vi "niFpga wdp fft streaming control chain.vi"(6 "enable":bool, 8 "enable 1":bool, 11 "input frame start":bool) -> (0 "frame start":bool, 1 "index=0?":bool, 2 "switch":bool[](array[boolean]), 3 "twiddle factors 1":T1(array[cluster]), 5 "twiddle factors":T1(array[cluster]))   [LabVIEW 2017]
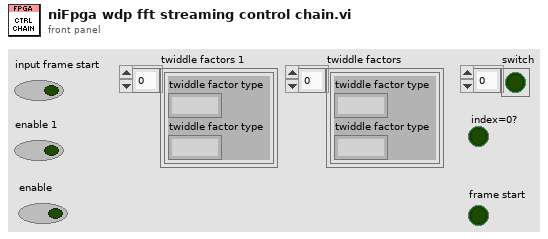
[diagram p1: front panel]
types:
  T1 = cluster{"twiddle factor type":fxp<+/-,16,2>, "twiddle factor type":fxp<+/-,16,2>}[]
  T2 = cluster{"twiddle factor type":fxp<+/-,16,2>, "twiddle factor type":fxp<+/-,16,2>}
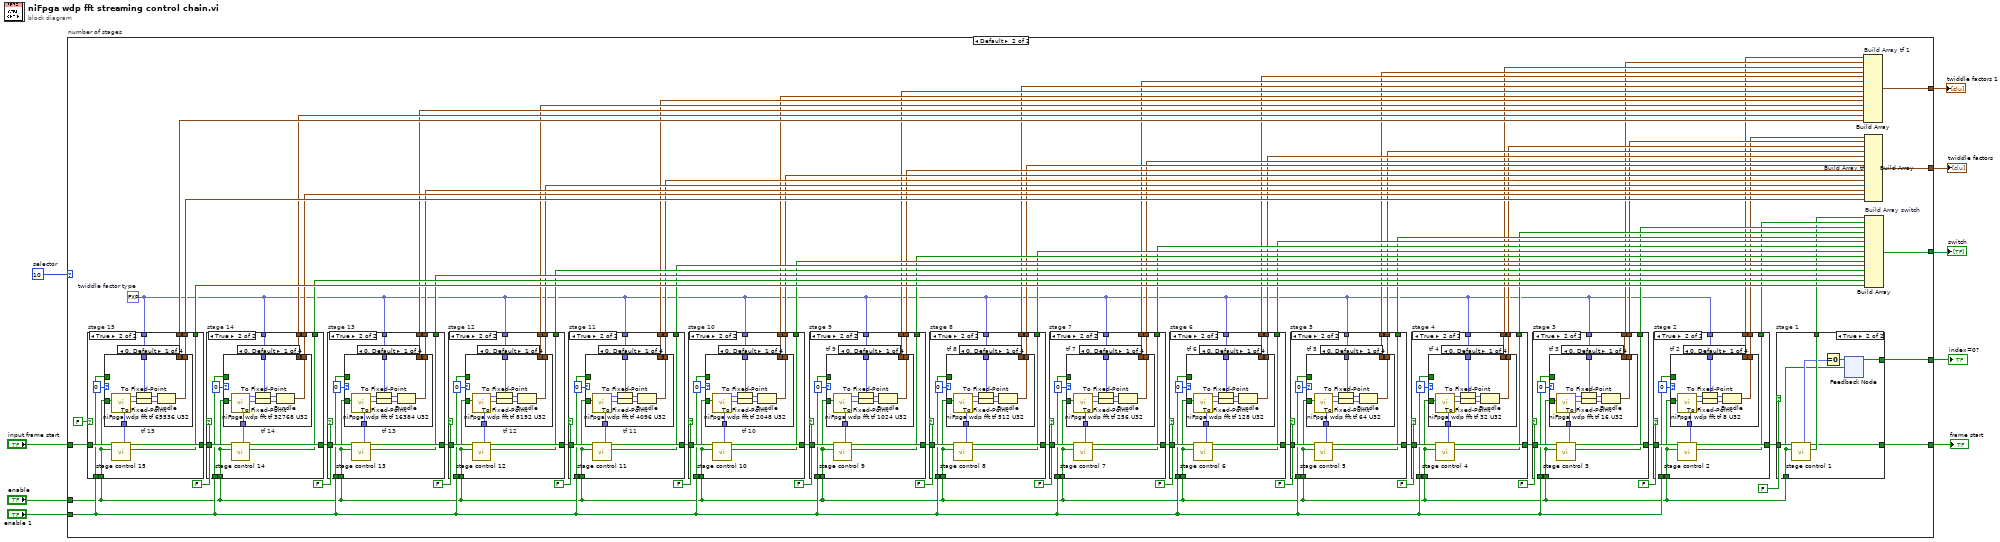
[diagram p0: block diagram]
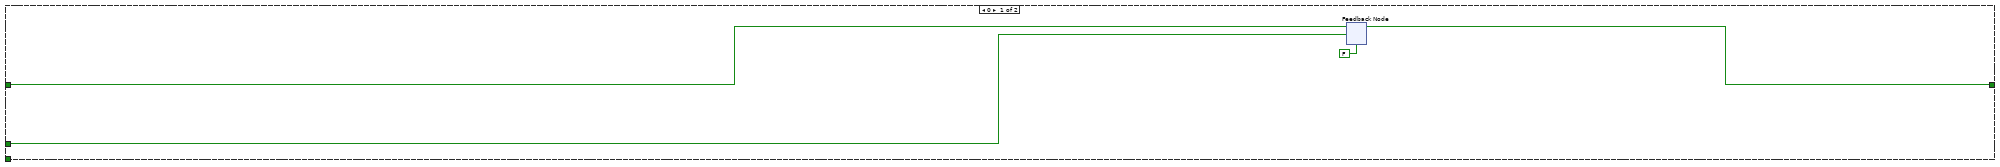
[diagram p2: hidden frame]
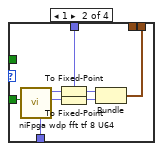
[diagram p5: hidden frame]
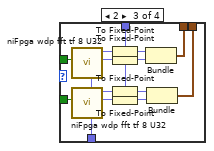
[diagram p6: hidden frame]
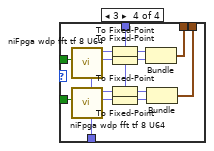
[diagram p7: hidden frame]
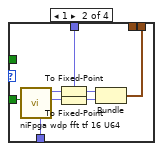
[diagram p9: hidden frame]
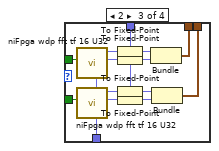
[diagram p10: hidden frame]
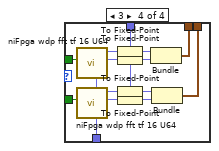
[diagram p11: hidden frame]
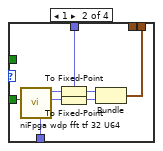
[diagram p13: hidden frame]
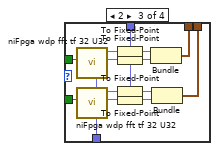
[diagram p14: hidden frame]
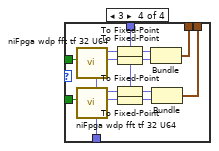
[diagram p15: hidden frame]
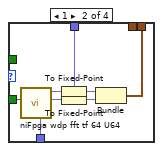
[diagram p17: hidden frame]
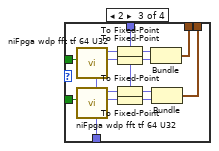
[diagram p18: hidden frame]
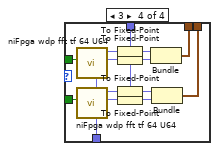
[diagram p19: hidden frame]
diagram:
  w2 = u8 10  # selector
  n1 = case "number of stages" shown="Default" w2 {
    tunnel: [_ w94] -> w9
    tunnel: [_ w93] -> w8
    tunnel: [_ w92] -> w7
    tunnel: "input frame start" -> [w12 w91]
    tunnel: [w11 w14] -> w5
    tunnel: "enable" -> [w10 w17]
    tunnel: "enable 1" -> [_ w35]
    tunnel: [_ w32] -> w1
    frame 0 {
      n2 = feedback #1(FALSE ("input frame start")) -> (w11:bool)
      n3 = feedback-in #1(w12, w10) -> ()
    }
    frame Default {
      w16 = fxp<+/-,16,2> 0.0  # twiddle factor type
      n4 = case "stage 15" shown="True" FALSE {
        tunnel: w91 -> [w818 w828]
        tunnel: [w818 w827] -> w87
        tunnel: w17 -> [_ w826]
        tunnel: w35 -> [_ w825]
        tunnel: [_ w824] -> w90
        tunnel: [_ w823] -> w89
        tunnel: [_ w822] -> w88
        tunnel: w16 -> [_ w819]
        frame False {
        }
        frame True {
          n5 = call "stage control 15"("enable"=w826, "frame start in"=w828) -> ("next switch"=w822:bool, "frame start out"=w827:bool, "twid index"=w820:fxp<+,15,15>)  [unwired: 7 in]
          n6 = case "tf 15" shown="0, Default" i16 0 {
            tunnel: w819 -> [w830 w838 w854 w868]
            tunnel: w826 -> [w834 w842 w853 w867]
            tunnel: w825 -> [_ _ w852 w866]
            tunnel: [_ _ w847 w861] -> w824
            tunnel: [w831 w839 w846 w860] -> w823
            tunnel: w820 -> [w829 w837 w845 w859]
            frame 0, Default {
              n7 = call <vilib>:"niFpga wdp fft tf 65536 U32.vi"("index"=w829, "enable"=w834) -> ("imag"=w835:fxp<+/-,16,2>, "real"=w836:fxp<+/-,16,2>)  [unwired: 8 in]
              n8 = To Fixed-Point(fixed-point type=w830, number=w836) -> (fixed-point=w833:fxp<+/-,16,2>)
              n9 = To Fixed-Point(fixed-point type=w830, number=w835) -> (fixed-point=w832:fxp<+/-,16,2>)
              n10 = Bundle("twiddle factor type"=w833, "twiddle factor type"=w832) -> (w831:T2)  [unwired: 1 in]
            }
            frame 1 {
              n11 = call <vilib>:"niFpga wdp fft tf 65536 U64.vi"("index"=w837, "enable"=w842) -> ("imag"=w843:fxp<+/-,32,2>, "real"=w844:fxp<+/-,32,2>)  [unwired: 8 in]
              n12 = To Fixed-Point(fixed-point type=w838, number=w844) -> (fixed-point=w841:fxp<+/-,16,2>)
              n13 = To Fixed-Point(fixed-point type=w838, number=w843) -> (fixed-point=w840:fxp<+/-,16,2>)
              n14 = Bundle("twiddle factor type"=w841, "twiddle factor type"=w840) -> (w839:T2)  [unwired: 1 in]
            }
            frame 2 {
              n15 = call <vilib>:"niFpga wdp fft tf 65536 U32.vi"("index"=w845, "enable"=w852) -> ("imag"=w856:fxp<+/-,16,2>, "real"=w857:fxp<+/-,16,2>)  [unwired: 8 in]
              n16 = call <vilib>:"niFpga wdp fft tf 65536 U32.vi"("index"=w845, "enable"=w853) -> ("imag"=w855:fxp<+/-,16,2>, "real"=w858:fxp<+/-,16,2>)  [unwired: 8 in]
              n17 = To Fixed-Point(fixed-point type=w854, number=w857) -> (fixed-point=w851:fxp<+/-,16,2>)
              n18 = To Fixed-Point(fixed-point type=w854, number=w856) -> (fixed-point=w850:fxp<+/-,16,2>)
              n19 = To Fixed-Point(fixed-point type=w854, number=w858) -> (fixed-point=w849:fxp<+/-,16,2>)
              n20 = To Fixed-Point(fixed-point type=w854, number=w855) -> (fixed-point=w848:fxp<+/-,16,2>)
              n21 = Bundle("twiddle factor type"=w851, "twiddle factor type"=w850) -> (w847:T2)  [unwired: 1 in]
              n22 = Bundle("twiddle factor type"=w849, "twiddle factor type"=w848) -> (w846:T2)  [unwired: 1 in]
            }
            frame 3 {
              n23 = call <vilib>:"niFpga wdp fft tf 65536 U64.vi"("index"=w859, "enable"=w866) -> ("imag"=w870:fxp<+/-,32,2>, "real"=w871:fxp<+/-,32,2>)  [unwired: 8 in]
              n24 = call <vilib>:"niFpga wdp fft tf 65536 U64.vi"("index"=w859, "enable"=w867) -> ("imag"=w869:fxp<+/-,32,2>, "real"=w872:fxp<+/-,32,2>)  [unwired: 8 in]
              n25 = To Fixed-Point(fixed-point type=w868, number=w871) -> (fixed-point=w865:fxp<+/-,16,2>)
              n26 = To Fixed-Point(fixed-point type=w868, number=w870) -> (fixed-point=w864:fxp<+/-,16,2>)
              n27 = To Fixed-Point(fixed-point type=w868, number=w872) -> (fixed-point=w863:fxp<+/-,16,2>)
              n28 = To Fixed-Point(fixed-point type=w868, number=w869) -> (fixed-point=w862:fxp<+/-,16,2>)
              n29 = Bundle("twiddle factor type"=w865, "twiddle factor type"=w864) -> (w861:T2)  [unwired: 1 in]
              n30 = Bundle("twiddle factor type"=w863, "twiddle factor type"=w862) -> (w860:T2)  [unwired: 1 in]
            }
          }
        }
      }
      n31 = case "stage 14" shown="True" FALSE {
        tunnel: w87 -> [w763 w773]
        tunnel: [w763 w772] -> w83
        tunnel: w17 -> [_ w771]
        tunnel: w35 -> [_ w770]
        tunnel: [_ w769] -> w86
        tunnel: [_ w768] -> w85
        tunnel: [_ w767] -> w84
        tunnel: w16 -> [_ w764]
        frame False {
        }
        frame True {
          n32 = call "stage control 14"("enable"=w771, "frame start in"=w773) -> ("next switch"=w767:bool, "frame start out"=w772:bool, "twid index"=w765:fxp<+,14,14>)  [unwired: 7 in]
          n33 = case "tf 14" shown="0, Default" i16 0 {
            tunnel: w764 -> [w775 w783 w799 w813]
            tunnel: w771 -> [w779 w787 w798 w812]
            tunnel: w770 -> [_ _ w797 w811]
            tunnel: [_ _ w792 w806] -> w769
            tunnel: [w776 w784 w791 w805] -> w768
            tunnel: w765 -> [w774 w782 w790 w804]
            frame 0, Default {
              n34 = call <vilib>:"niFpga wdp fft tf 32768 U32.vi"("index"=w774, "enable"=w779) -> ("imag"=w780:fxp<+/-,16,2>, "real"=w781:fxp<+/-,16,2>)  [unwired: 8 in]
              n35 = To Fixed-Point(fixed-point type=w775, number=w781) -> (fixed-point=w778:fxp<+/-,16,2>)
              n36 = To Fixed-Point(fixed-point type=w775, number=w780) -> (fixed-point=w777:fxp<+/-,16,2>)
              n37 = Bundle("twiddle factor type"=w778, "twiddle factor type"=w777) -> (w776:T2)  [unwired: 1 in]
            }
            frame 1 {
              n38 = call <vilib>:"niFpga wdp fft tf 32768 U64.vi"("index"=w782, "enable"=w787) -> ("imag"=w788:fxp<+/-,32,2>, "real"=w789:fxp<+/-,32,2>)  [unwired: 8 in]
              n39 = To Fixed-Point(fixed-point type=w783, number=w789) -> (fixed-point=w786:fxp<+/-,16,2>)
              n40 = To Fixed-Point(fixed-point type=w783, number=w788) -> (fixed-point=w785:fxp<+/-,16,2>)
              n41 = Bundle("twiddle factor type"=w786, "twiddle factor type"=w785) -> (w784:T2)  [unwired: 1 in]
            }
            frame 2 {
              n42 = call <vilib>:"niFpga wdp fft tf 32768 U32.vi"("index"=w790, "enable"=w797) -> ("imag"=w801:fxp<+/-,16,2>, "real"=w802:fxp<+/-,16,2>)  [unwired: 8 in]
              n43 = call <vilib>:"niFpga wdp fft tf 32768 U32.vi"("index"=w790, "enable"=w798) -> ("imag"=w800:fxp<+/-,16,2>, "real"=w803:fxp<+/-,16,2>)  [unwired: 8 in]
              n44 = To Fixed-Point(fixed-point type=w799, number=w802) -> (fixed-point=w796:fxp<+/-,16,2>)
              n45 = To Fixed-Point(fixed-point type=w799, number=w801) -> (fixed-point=w795:fxp<+/-,16,2>)
              n46 = To Fixed-Point(fixed-point type=w799, number=w803) -> (fixed-point=w794:fxp<+/-,16,2>)
              n47 = To Fixed-Point(fixed-point type=w799, number=w800) -> (fixed-point=w793:fxp<+/-,16,2>)
              n48 = Bundle("twiddle factor type"=w796, "twiddle factor type"=w795) -> (w792:T2)  [unwired: 1 in]
              n49 = Bundle("twiddle factor type"=w794, "twiddle factor type"=w793) -> (w791:T2)  [unwired: 1 in]
            }
            frame 3 {
              n50 = call <vilib>:"niFpga wdp fft tf 32768 U64.vi"("index"=w804, "enable"=w811) -> ("imag"=w815:fxp<+/-,32,2>, "real"=w816:fxp<+/-,32,2>)  [unwired: 8 in]
              n51 = call <vilib>:"niFpga wdp fft tf 32768 U64.vi"("index"=w804, "enable"=w812) -> ("imag"=w814:fxp<+/-,32,2>, "real"=w817:fxp<+/-,32,2>)  [unwired: 8 in]
              n52 = To Fixed-Point(fixed-point type=w813, number=w816) -> (fixed-point=w810:fxp<+/-,16,2>)
              n53 = To Fixed-Point(fixed-point type=w813, number=w815) -> (fixed-point=w809:fxp<+/-,16,2>)
              n54 = To Fixed-Point(fixed-point type=w813, number=w817) -> (fixed-point=w808:fxp<+/-,16,2>)
              n55 = To Fixed-Point(fixed-point type=w813, number=w814) -> (fixed-point=w807:fxp<+/-,16,2>)
              n56 = Bundle("twiddle factor type"=w810, "twiddle factor type"=w809) -> (w806:T2)  [unwired: 1 in]
              n57 = Bundle("twiddle factor type"=w808, "twiddle factor type"=w807) -> (w805:T2)  [unwired: 1 in]
            }
          }
        }
      }
      n58 = case "stage 13" shown="True" FALSE {
        tunnel: w83 -> [w708 w718]
        tunnel: [w708 w717] -> w79
        tunnel: w17 -> [_ w716]
        tunnel: w35 -> [_ w715]
        tunnel: [_ w714] -> w82
        tunnel: [_ w713] -> w81
        tunnel: [_ w712] -> w80
        tunnel: w16 -> [_ w709]
        frame False {
        }
        frame True {
          n59 = call "stage control 13"("enable"=w716, "frame start in"=w718) -> ("next switch"=w712:bool, "frame start out"=w717:bool, "twid index"=w710:fxp<+,13,13>)  [unwired: 7 in]
          n60 = case "tf 13" shown="0, Default" i16 0 {
            tunnel: w709 -> [w720 w728 w744 w758]
            tunnel: w716 -> [w724 w732 w743 w757]
            tunnel: w715 -> [_ _ w742 w756]
            tunnel: [_ _ w737 w751] -> w714
            tunnel: [w721 w729 w736 w750] -> w713
            tunnel: w710 -> [w719 w727 w735 w749]
            frame 0, Default {
              n61 = call <vilib>:"niFpga wdp fft tf 16384 U32.vi"("index"=w719, "enable"=w724) -> ("imag"=w725:fxp<+/-,16,2>, "real"=w726:fxp<+/-,16,2>)  [unwired: 8 in]
              n62 = To Fixed-Point(fixed-point type=w720, number=w726) -> (fixed-point=w723:fxp<+/-,16,2>)
              n63 = To Fixed-Point(fixed-point type=w720, number=w725) -> (fixed-point=w722:fxp<+/-,16,2>)
              n64 = Bundle("twiddle factor type"=w723, "twiddle factor type"=w722) -> (w721:T2)  [unwired: 1 in]
            }
            frame 1 {
              n65 = call <vilib>:"niFpga wdp fft tf 16384 U64.vi"("index"=w727, "enable"=w732) -> ("imag"=w733:fxp<+/-,32,2>, "real"=w734:fxp<+/-,32,2>)  [unwired: 8 in]
              n66 = To Fixed-Point(fixed-point type=w728, number=w734) -> (fixed-point=w731:fxp<+/-,16,2>)
              n67 = To Fixed-Point(fixed-point type=w728, number=w733) -> (fixed-point=w730:fxp<+/-,16,2>)
              n68 = Bundle("twiddle factor type"=w731, "twiddle factor type"=w730) -> (w729:T2)  [unwired: 1 in]
            }
            frame 2 {
              n69 = call <vilib>:"niFpga wdp fft tf 16384 U32.vi"("index"=w735, "enable"=w742) -> ("imag"=w746:fxp<+/-,16,2>, "real"=w747:fxp<+/-,16,2>)  [unwired: 8 in]
              n70 = call <vilib>:"niFpga wdp fft tf 16384 U32.vi"("index"=w735, "enable"=w743) -> ("imag"=w745:fxp<+/-,16,2>, "real"=w748:fxp<+/-,16,2>)  [unwired: 8 in]
              n71 = To Fixed-Point(fixed-point type=w744, number=w747) -> (fixed-point=w741:fxp<+/-,16,2>)
              n72 = To Fixed-Point(fixed-point type=w744, number=w746) -> (fixed-point=w740:fxp<+/-,16,2>)
              n73 = To Fixed-Point(fixed-point type=w744, number=w748) -> (fixed-point=w739:fxp<+/-,16,2>)
              n74 = To Fixed-Point(fixed-point type=w744, number=w745) -> (fixed-point=w738:fxp<+/-,16,2>)
              n75 = Bundle("twiddle factor type"=w741, "twiddle factor type"=w740) -> (w737:T2)  [unwired: 1 in]
              n76 = Bundle("twiddle factor type"=w739, "twiddle factor type"=w738) -> (w736:T2)  [unwired: 1 in]
            }
            frame 3 {
              n77 = call <vilib>:"niFpga wdp fft tf 16384 U64.vi"("index"=w749, "enable"=w756) -> ("imag"=w760:fxp<+/-,32,2>, "real"=w761:fxp<+/-,32,2>)  [unwired: 8 in]
              n78 = call <vilib>:"niFpga wdp fft tf 16384 U64.vi"("index"=w749, "enable"=w757) -> ("imag"=w759:fxp<+/-,32,2>, "real"=w762:fxp<+/-,32,2>)  [unwired: 8 in]
              n79 = To Fixed-Point(fixed-point type=w758, number=w761) -> (fixed-point=w755:fxp<+/-,16,2>)
              n80 = To Fixed-Point(fixed-point type=w758, number=w760) -> (fixed-point=w754:fxp<+/-,16,2>)
              n81 = To Fixed-Point(fixed-point type=w758, number=w762) -> (fixed-point=w753:fxp<+/-,16,2>)
              n82 = To Fixed-Point(fixed-point type=w758, number=w759) -> (fixed-point=w752:fxp<+/-,16,2>)
              n83 = Bundle("twiddle factor type"=w755, "twiddle factor type"=w754) -> (w751:T2)  [unwired: 1 in]
              n84 = Bundle("twiddle factor type"=w753, "twiddle factor type"=w752) -> (w750:T2)  [unwired: 1 in]
            }
          }
        }
      }
      n85 = case "stage 12" shown="True" FALSE {
        tunnel: w79 -> [w653 w663]
        tunnel: [w653 w662] -> w75
        tunnel: w17 -> [_ w661]
        tunnel: w35 -> [_ w660]
        tunnel: [_ w659] -> w78
        tunnel: [_ w658] -> w77
        tunnel: [_ w657] -> w76
        tunnel: w16 -> [_ w654]
        frame False {
        }
        frame True {
          n86 = call "stage control 12"("enable"=w661, "frame start in"=w663) -> ("next switch"=w657:bool, "frame start out"=w662:bool, "twid index"=w655:fxp<+,12,12>)  [unwired: 7 in]
          n87 = case "tf 12" shown="0, Default" i16 0 {
            tunnel: w654 -> [w665 w673 w689 w703]
            tunnel: w661 -> [w669 w677 w688 w702]
            tunnel: w660 -> [_ _ w687 w701]
            tunnel: [_ _ w682 w696] -> w659
            tunnel: [w666 w674 w681 w695] -> w658
            tunnel: w655 -> [w664 w672 w680 w694]
            frame 0, Default {
              n88 = call <vilib>:"niFpga wdp fft tf 8192 U32.vi"("index"=w664, "enable"=w669) -> ("imag"=w670:fxp<+/-,16,2>, "real"=w671:fxp<+/-,16,2>)  [unwired: 8 in]
              n89 = To Fixed-Point(fixed-point type=w665, number=w671) -> (fixed-point=w668:fxp<+/-,16,2>)
              n90 = To Fixed-Point(fixed-point type=w665, number=w670) -> (fixed-point=w667:fxp<+/-,16,2>)
              n91 = Bundle("twiddle factor type"=w668, "twiddle factor type"=w667) -> (w666:T2)  [unwired: 1 in]
            }
            frame 1 {
              n92 = call <vilib>:"niFpga wdp fft tf 8192 U64.vi"("index"=w672, "enable"=w677) -> ("imag"=w678:fxp<+/-,32,2>, "real"=w679:fxp<+/-,32,2>)  [unwired: 8 in]
              n93 = To Fixed-Point(fixed-point type=w673, number=w679) -> (fixed-point=w676:fxp<+/-,16,2>)
              n94 = To Fixed-Point(fixed-point type=w673, number=w678) -> (fixed-point=w675:fxp<+/-,16,2>)
              n95 = Bundle("twiddle factor type"=w676, "twiddle factor type"=w675) -> (w674:T2)  [unwired: 1 in]
            }
            frame 2 {
              n96 = call <vilib>:"niFpga wdp fft tf 8192 U32.vi"("index"=w680, "enable"=w687) -> ("imag"=w691:fxp<+/-,16,2>, "real"=w692:fxp<+/-,16,2>)  [unwired: 8 in]
              n97 = call <vilib>:"niFpga wdp fft tf 8192 U32.vi"("index"=w680, "enable"=w688) -> ("imag"=w690:fxp<+/-,16,2>, "real"=w693:fxp<+/-,16,2>)  [unwired: 8 in]
              n98 = To Fixed-Point(fixed-point type=w689, number=w692) -> (fixed-point=w686:fxp<+/-,16,2>)
              n99 = To Fixed-Point(fixed-point type=w689, number=w691) -> (fixed-point=w685:fxp<+/-,16,2>)
              n100 = To Fixed-Point(fixed-point type=w689, number=w693) -> (fixed-point=w684:fxp<+/-,16,2>)
              n101 = To Fixed-Point(fixed-point type=w689, number=w690) -> (fixed-point=w683:fxp<+/-,16,2>)
              n102 = Bundle("twiddle factor type"=w686, "twiddle factor type"=w685) -> (w682:T2)  [unwired: 1 in]
              n103 = Bundle("twiddle factor type"=w684, "twiddle factor type"=w683) -> (w681:T2)  [unwired: 1 in]
            }
            frame 3 {
              n104 = call <vilib>:"niFpga wdp fft tf 8192 U64.vi"("index"=w694, "enable"=w701) -> ("imag"=w705:fxp<+/-,32,2>, "real"=w706:fxp<+/-,32,2>)  [unwired: 8 in]
              n105 = call <vilib>:"niFpga wdp fft tf 8192 U64.vi"("index"=w694, "enable"=w702) -> ("imag"=w704:fxp<+/-,32,2>, "real"=w707:fxp<+/-,32,2>)  [unwired: 8 in]
              n106 = To Fixed-Point(fixed-point type=w703, number=w706) -> (fixed-point=w700:fxp<+/-,16,2>)
              n107 = To Fixed-Point(fixed-point type=w703, number=w705) -> (fixed-point=w699:fxp<+/-,16,2>)
              n108 = To Fixed-Point(fixed-point type=w703, number=w707) -> (fixed-point=w698:fxp<+/-,16,2>)
              n109 = To Fixed-Point(fixed-point type=w703, number=w704) -> (fixed-point=w697:fxp<+/-,16,2>)
              n110 = Bundle("twiddle factor type"=w700, "twiddle factor type"=w699) -> (w696:T2)  [unwired: 1 in]
              n111 = Bundle("twiddle factor type"=w698, "twiddle factor type"=w697) -> (w695:T2)  [unwired: 1 in]
            }
          }
        }
      }
      n112 = case "stage 11" shown="True" FALSE {
        tunnel: w75 -> [w598 w608]
        tunnel: [w598 w607] -> w71
        tunnel: w17 -> [_ w606]
        tunnel: w35 -> [_ w605]
        tunnel: [_ w604] -> w74
        tunnel: [_ w603] -> w73
        tunnel: [_ w602] -> w72
        tunnel: w16 -> [_ w599]
        frame False {
        }
        frame True {
          n113 = call "stage control 11"("enable"=w606, "frame start in"=w608) -> ("next switch"=w602:bool, "frame start out"=w607:bool, "twid index"=w600:fxp<+,11,11>)  [unwired: 7 in]
          n114 = case "tf 11" shown="0, Default" i16 0 {
            tunnel: w599 -> [w610 w618 w634 w648]
            tunnel: w606 -> [w614 w622 w633 w647]
            tunnel: w605 -> [_ _ w632 w646]
            tunnel: [_ _ w627 w641] -> w604
            tunnel: [w611 w619 w626 w640] -> w603
            tunnel: w600 -> [w609 w617 w625 w639]
            frame 0, Default {
              n115 = call <vilib>:"niFpga wdp fft tf 4096 U32.vi"("index"=w609, "enable"=w614) -> ("imag"=w615:fxp<+/-,16,2>, "real"=w616:fxp<+/-,16,2>)  [unwired: 8 in]
              n116 = To Fixed-Point(fixed-point type=w610, number=w616) -> (fixed-point=w613:fxp<+/-,16,2>)
              n117 = To Fixed-Point(fixed-point type=w610, number=w615) -> (fixed-point=w612:fxp<+/-,16,2>)
              n118 = Bundle("twiddle factor type"=w613, "twiddle factor type"=w612) -> (w611:T2)  [unwired: 1 in]
            }
            frame 1 {
              n119 = call <vilib>:"niFpga wdp fft tf 4096 U64.vi"("index"=w617, "enable"=w622) -> ("imag"=w623:fxp<+/-,32,2>, "real"=w624:fxp<+/-,32,2>)  [unwired: 8 in]
              n120 = To Fixed-Point(fixed-point type=w618, number=w624) -> (fixed-point=w621:fxp<+/-,16,2>)
              n121 = To Fixed-Point(fixed-point type=w618, number=w623) -> (fixed-point=w620:fxp<+/-,16,2>)
              n122 = Bundle("twiddle factor type"=w621, "twiddle factor type"=w620) -> (w619:T2)  [unwired: 1 in]
            }
            frame 2 {
              n123 = call <vilib>:"niFpga wdp fft tf 4096 U32.vi"("index"=w625, "enable"=w632) -> ("imag"=w636:fxp<+/-,16,2>, "real"=w637:fxp<+/-,16,2>)  [unwired: 8 in]
              n124 = call <vilib>:"niFpga wdp fft tf 4096 U32.vi"("index"=w625, "enable"=w633) -> ("imag"=w635:fxp<+/-,16,2>, "real"=w638:fxp<+/-,16,2>)  [unwired: 8 in]
              n125 = To Fixed-Point(fixed-point type=w634, number=w637) -> (fixed-point=w631:fxp<+/-,16,2>)
              n126 = To Fixed-Point(fixed-point type=w634, number=w636) -> (fixed-point=w630:fxp<+/-,16,2>)
              n127 = To Fixed-Point(fixed-point type=w634, number=w638) -> (fixed-point=w629:fxp<+/-,16,2>)
              n128 = To Fixed-Point(fixed-point type=w634, number=w635) -> (fixed-point=w628:fxp<+/-,16,2>)
              n129 = Bundle("twiddle factor type"=w631, "twiddle factor type"=w630) -> (w627:T2)  [unwired: 1 in]
              n130 = Bundle("twiddle factor type"=w629, "twiddle factor type"=w628) -> (w626:T2)  [unwired: 1 in]
            }
            frame 3 {
              n131 = call <vilib>:"niFpga wdp fft tf 4096 U64.vi"("index"=w639, "enable"=w646) -> ("imag"=w650:fxp<+/-,32,2>, "real"=w651:fxp<+/-,32,2>)  [unwired: 8 in]
              n132 = call <vilib>:"niFpga wdp fft tf 4096 U64.vi"("index"=w639, "enable"=w647) -> ("imag"=w649:fxp<+/-,32,2>, "real"=w652:fxp<+/-,32,2>)  [unwired: 8 in]
              n133 = To Fixed-Point(fixed-point type=w648, number=w651) -> (fixed-point=w645:fxp<+/-,16,2>)
              n134 = To Fixed-Point(fixed-point type=w648, number=w650) -> (fixed-point=w644:fxp<+/-,16,2>)
              n135 = To Fixed-Point(fixed-point type=w648, number=w652) -> (fixed-point=w643:fxp<+/-,16,2>)
              n136 = To Fixed-Point(fixed-point type=w648, number=w649) -> (fixed-point=w642:fxp<+/-,16,2>)
              n137 = Bundle("twiddle factor type"=w645, "twiddle factor type"=w644) -> (w641:T2)  [unwired: 1 in]
              n138 = Bundle("twiddle factor type"=w643, "twiddle factor type"=w642) -> (w640:T2)  [unwired: 1 in]
            }
          }
        }
      }
      n139 = case "stage 10" shown="True" FALSE {
        tunnel: w71 -> [w543 w553]
        tunnel: [w543 w552] -> w67
        tunnel: w17 -> [_ w551]
        tunnel: w35 -> [_ w550]
        tunnel: [_ w549] -> w70
        tunnel: [_ w548] -> w69
        tunnel: [_ w547] -> w68
        tunnel: w16 -> [_ w544]
        frame False {
        }
        frame True {
          n140 = call "stage control 10"("enable"=w551, "frame start in"=w553) -> ("next switch"=w547:bool, "frame start out"=w552:bool, "twid index"=w545:fxp<+,10,10>)  [unwired: 7 in]
          n141 = case "tf 10" shown="0, Default" i16 0 {
            tunnel: w544 -> [w555 w563 w579 w593]
            tunnel: w551 -> [w559 w567 w578 w592]
            tunnel: w550 -> [_ _ w577 w591]
            tunnel: [_ _ w572 w586] -> w549
            tunnel: [w556 w564 w571 w585] -> w548
            tunnel: w545 -> [w554 w562 w570 w584]
            frame 0, Default {
              n142 = call <vilib>:"niFpga wdp fft tf 2048 U32.vi"("index"=w554, "enable"=w559) -> ("imag"=w560:fxp<+/-,16,2>, "real"=w561:fxp<+/-,16,2>)  [unwired: 8 in]
              n143 = To Fixed-Point(fixed-point type=w555, number=w561) -> (fixed-point=w558:fxp<+/-,16,2>)
              n144 = To Fixed-Point(fixed-point type=w555, number=w560) -> (fixed-point=w557:fxp<+/-,16,2>)
              n145 = Bundle("twiddle factor type"=w558, "twiddle factor type"=w557) -> (w556:T2)  [unwired: 1 in]
            }
            frame 1 {
              n146 = call <vilib>:"niFpga wdp fft tf 2048 U64.vi"("index"=w562, "enable"=w567) -> ("imag"=w568:fxp<+/-,32,2>, "real"=w569:fxp<+/-,32,2>)  [unwired: 8 in]
              n147 = To Fixed-Point(fixed-point type=w563, number=w569) -> (fixed-point=w566:fxp<+/-,16,2>)
              n148 = To Fixed-Point(fixed-point type=w563, number=w568) -> (fixed-point=w565:fxp<+/-,16,2>)
              n149 = Bundle("twiddle factor type"=w566, "twiddle factor type"=w565) -> (w564:T2)  [unwired: 1 in]
            }
            frame 2 {
              n150 = call <vilib>:"niFpga wdp fft tf 2048 U32.vi"("index"=w570, "enable"=w577) -> ("imag"=w581:fxp<+/-,16,2>, "real"=w582:fxp<+/-,16,2>)  [unwired: 8 in]
              n151 = call <vilib>:"niFpga wdp fft tf 2048 U32.vi"("index"=w570, "enable"=w578) -> ("imag"=w580:fxp<+/-,16,2>, "real"=w583:fxp<+/-,16,2>)  [unwired: 8 in]
              n152 = To Fixed-Point(fixed-point type=w579, number=w582) -> (fixed-point=w576:fxp<+/-,16,2>)
              n153 = To Fixed-Point(fixed-point type=w579, number=w581) -> (fixed-point=w575:fxp<+/-,16,2>)
              n154 = To Fixed-Point(fixed-point type=w579, number=w583) -> (fixed-point=w574:fxp<+/-,16,2>)
              n155 = To Fixed-Point(fixed-point type=w579, number=w580) -> (fixed-point=w573:fxp<+/-,16,2>)
              n156 = Bundle("twiddle factor type"=w576, "twiddle factor type"=w575) -> (w572:T2)  [unwired: 1 in]
              n157 = Bundle("twiddle factor type"=w574, "twiddle factor type"=w573) -> (w571:T2)  [unwired: 1 in]
            }
            frame 3 {
              n158 = call <vilib>:"niFpga wdp fft tf 2048 U64.vi"("index"=w584, "enable"=w591) -> ("imag"=w595:fxp<+/-,32,2>, "real"=w596:fxp<+/-,32,2>)  [unwired: 8 in]
              n159 = call <vilib>:"niFpga wdp fft tf 2048 U64.vi"("index"=w584, "enable"=w592) -> ("imag"=w594:fxp<+/-,32,2>, "real"=w597:fxp<+/-,32,2>)  [unwired: 8 in]
              n160 = To Fixed-Point(fixed-point type=w593, number=w596) -> (fixed-point=w590:fxp<+/-,16,2>)
              n161 = To Fixed-Point(fixed-point type=w593, number=w595) -> (fixed-point=w589:fxp<+/-,16,2>)
              n162 = To Fixed-Point(fixed-point type=w593, number=w597) -> (fixed-point=w588:fxp<+/-,16,2>)
              n163 = To Fixed-Point(fixed-point type=w593, number=w594) -> (fixed-point=w587:fxp<+/-,16,2>)
              n164 = Bundle("twiddle factor type"=w590, "twiddle factor type"=w589) -> (w586:T2)  [unwired: 1 in]
              n165 = Bundle("twiddle factor type"=w588, "twiddle factor type"=w587) -> (w585:T2)  [unwired: 1 in]
            }
          }
        }
      }
      n166 = case "stage 9" shown="True" FALSE {
        tunnel: w67 -> [w488 w498]
        tunnel: [w488 w497] -> w63
        tunnel: w17 -> [_ w496]
        tunnel: w35 -> [_ w495]
        tunnel: [_ w494] -> w66
        tunnel: [_ w493] -> w65
        tunnel: [_ w492] -> w64
        tunnel: w16 -> [_ w489]
        frame False {
        }
        frame True {
          n167 = call "stage control 9"("enable"=w496, "frame start in"=w498) -> ("next switch"=w492:bool, "frame start out"=w497:bool, "twid index"=w490:fxp<+,9,9>)  [unwired: 7 in]
          n168 = case "tf 9" shown="0, Default" i16 0 {
            tunnel: w489 -> [w500 w508 w524 w538]
            tunnel: w496 -> [w504 w512 w523 w537]
            tunnel: w495 -> [_ _ w522 w536]
            tunnel: [_ _ w517 w531] -> w494
            tunnel: [w501 w509 w516 w530] -> w493
            tunnel: w490 -> [w499 w507 w515 w529]
            frame 0, Default {
              n169 = call <vilib>:"niFpga wdp fft tf 1024 U32.vi"("index"=w499, "enable"=w504) -> ("imag"=w505:fxp<+/-,16,2>, "real"=w506:fxp<+/-,16,2>)  [unwired: 8 in]
              n170 = To Fixed-Point(fixed-point type=w500, number=w506) -> (fixed-point=w503:fxp<+/-,16,2>)
              n171 = To Fixed-Point(fixed-point type=w500, number=w505) -> (fixed-point=w502:fxp<+/-,16,2>)
              n172 = Bundle("twiddle factor type"=w503, "twiddle factor type"=w502) -> (w501:T2)  [unwired: 1 in]
            }
            frame 1 {
              n173 = call <vilib>:"niFpga wdp fft tf 1024 U64.vi"("index"=w507, "enable"=w512) -> ("imag"=w513:fxp<+/-,32,2>, "real"=w514:fxp<+/-,32,2>)  [unwired: 8 in]
              n174 = To Fixed-Point(fixed-point type=w508, number=w514) -> (fixed-point=w511:fxp<+/-,16,2>)
              n175 = To Fixed-Point(fixed-point type=w508, number=w513) -> (fixed-point=w510:fxp<+/-,16,2>)
              n176 = Bundle("twiddle factor type"=w511, "twiddle factor type"=w510) -> (w509:T2)  [unwired: 1 in]
            }
            frame 2 {
              n177 = call <vilib>:"niFpga wdp fft tf 1024 U32.vi"("index"=w515, "enable"=w522) -> ("imag"=w526:fxp<+/-,16,2>, "real"=w527:fxp<+/-,16,2>)  [unwired: 8 in]
              n178 = call <vilib>:"niFpga wdp fft tf 1024 U32.vi"("index"=w515, "enable"=w523) -> ("imag"=w525:fxp<+/-,16,2>, "real"=w528:fxp<+/-,16,2>)  [unwired: 8 in]
              n179 = To Fixed-Point(fixed-point type=w524, number=w527) -> (fixed-point=w521:fxp<+/-,16,2>)
              n180 = To Fixed-Point(fixed-point type=w524, number=w526) -> (fixed-point=w520:fxp<+/-,16,2>)
              n181 = To Fixed-Point(fixed-point type=w524, number=w528) -> (fixed-point=w519:fxp<+/-,16,2>)
              n182 = To Fixed-Point(fixed-point type=w524, number=w525) -> (fixed-point=w518:fxp<+/-,16,2>)
              n183 = Bundle("twiddle factor type"=w521, "twiddle factor type"=w520) -> (w517:T2)  [unwired: 1 in]
              n184 = Bundle("twiddle factor type"=w519, "twiddle factor type"=w518) -> (w516:T2)  [unwired: 1 in]
            }
            frame 3 {
              n185 = call <vilib>:"niFpga wdp fft tf 1024 U64.vi"("index"=w529, "enable"=w536) -> ("imag"=w540:fxp<+/-,32,2>, "real"=w541:fxp<+/-,32,2>)  [unwired: 8 in]
              n186 = call <vilib>:"niFpga wdp fft tf 1024 U64.vi"("index"=w529, "enable"=w537) -> ("imag"=w539:fxp<+/-,32,2>, "real"=w542:fxp<+/-,32,2>)  [unwired: 8 in]
              n187 = To Fixed-Point(fixed-point type=w538, number=w541) -> (fixed-point=w535:fxp<+/-,16,2>)
              n188 = To Fixed-Point(fixed-point type=w538, number=w540) -> (fixed-point=w534:fxp<+/-,16,2>)
              n189 = To Fixed-Point(fixed-point type=w538, number=w542) -> (fixed-point=w533:fxp<+/-,16,2>)
              n190 = To Fixed-Point(fixed-point type=w538, number=w539) -> (fixed-point=w532:fxp<+/-,16,2>)
              n191 = Bundle("twiddle factor type"=w535, "twiddle factor type"=w534) -> (w531:T2)  [unwired: 1 in]
              n192 = Bundle("twiddle factor type"=w533, "twiddle factor type"=w532) -> (w530:T2)  [unwired: 1 in]
            }
          }
        }
      }
      n193 = case "stage 8" shown="True" FALSE {
        tunnel: w63 -> [w433 w443]
        tunnel: [w433 w442] -> w59
        tunnel: w17 -> [_ w441]
        tunnel: w35 -> [_ w440]
        tunnel: [_ w439] -> w62
        tunnel: [_ w438] -> w61
        tunnel: [_ w437] -> w60
        tunnel: w16 -> [_ w434]
        frame False {
        }
        frame True {
          n194 = call "stage control 8"("enable"=w441, "frame start in"=w443) -> ("next switch"=w437:bool, "frame start out"=w442:bool, "twid index"=w435:fxp<+,8,8>)  [unwired: 7 in]
          n195 = case "tf 8" shown="0, Default" i16 0 {
            tunnel: w434 -> [w445 w453 w469 w483]
            tunnel: w441 -> [w449 w457 w468 w482]
            tunnel: w440 -> [_ _ w467 w481]
            tunnel: [_ _ w462 w476] -> w439
            tunnel: [w446 w454 w461 w475] -> w438
            tunnel: w435 -> [w444 w452 w460 w474]
            frame 0, Default {
              n196 = call <vilib>:"niFpga wdp fft tf 512 U32.vi"("index"=w444, "enable"=w449) -> ("imag"=w450:fxp<+/-,16,2>, "real"=w451:fxp<+/-,16,2>)  [unwired: 8 in]
              n197 = To Fixed-Point(fixed-point type=w445, number=w451) -> (fixed-point=w448:fxp<+/-,16,2>)
              n198 = To Fixed-Point(fixed-point type=w445, number=w450) -> (fixed-point=w447:fxp<+/-,16,2>)
              n199 = Bundle("twiddle factor type"=w448, "twiddle factor type"=w447) -> (w446:T2)  [unwired: 1 in]
            }
            frame 1 {
              n200 = call <vilib>:"niFpga wdp fft tf 512 U64.vi"("index"=w452, "enable"=w457) -> ("imag"=w458:fxp<+/-,32,2>, "real"=w459:fxp<+/-,32,2>)  [unwired: 8 in]
              n201 = To Fixed-Point(fixed-point type=w453, number=w459) -> (fixed-point=w456:fxp<+/-,16,2>)
              n202 = To Fixed-Point(fixed-point type=w453, number=w458) -> (fixed-point=w455:fxp<+/-,16,2>)
              n203 = Bundle("twiddle factor type"=w456, "twiddle factor type"=w455) -> (w454:T2)  [unwired: 1 in]
            }
            frame 2 {
              n204 = call <vilib>:"niFpga wdp fft tf 512 U32.vi"("index"=w460, "enable"=w467) -> ("imag"=w471:fxp<+/-,16,2>, "real"=w472:fxp<+/-,16,2>)  [unwired: 8 in]
              n205 = call <vilib>:"niFpga wdp fft tf 512 U32.vi"("index"=w460, "enable"=w468) -> ("imag"=w470:fxp<+/-,16,2>, "real"=w473:fxp<+/-,16,2>)  [unwired: 8 in]
              n206 = To Fixed-Point(fixed-point type=w469, number=w472) -> (fixed-point=w466:fxp<+/-,16,2>)
              n207 = To Fixed-Point(fixed-point type=w469, number=w471) -> (fixed-point=w465:fxp<+/-,16,2>)
              n208 = To Fixed-Point(fixed-point type=w469, number=w473) -> (fixed-point=w464:fxp<+/-,16,2>)
              n209 = To Fixed-Point(fixed-point type=w469, number=w470) -> (fixed-point=w463:fxp<+/-,16,2>)
              n210 = Bundle("twiddle factor type"=w466, "twiddle factor type"=w465) -> (w462:T2)  [unwired: 1 in]
              n211 = Bundle("twiddle factor type"=w464, "twiddle factor type"=w463) -> (w461:T2)  [unwired: 1 in]
            }
            frame 3 {
              n212 = call <vilib>:"niFpga wdp fft tf 512 U64.vi"("index"=w474, "enable"=w481) -> ("imag"=w485:fxp<+/-,32,2>, "real"=w486:fxp<+/-,32,2>)  [unwired: 8 in]
              n213 = call <vilib>:"niFpga wdp fft tf 512 U64.vi"("index"=w474, "enable"=w482) -> ("imag"=w484:fxp<+/-,32,2>, "real"=w487:fxp<+/-,32,2>)  [unwired: 8 in]
              n214 = To Fixed-Point(fixed-point type=w483, number=w486) -> (fixed-point=w480:fxp<+/-,16,2>)
              n215 = To Fixed-Point(fixed-point type=w483, number=w485) -> (fixed-point=w479:fxp<+/-,16,2>)
              n216 = To Fixed-Point(fixed-point type=w483, number=w487) -> (fixed-point=w478:fxp<+/-,16,2>)
              n217 = To Fixed-Point(fixed-point type=w483, number=w484) -> (fixed-point=w477:fxp<+/-,16,2>)
              n218 = Bundle("twiddle factor type"=w480, "twiddle factor type"=w479) -> (w476:T2)  [unwired: 1 in]
              n219 = Bundle("twiddle factor type"=w478, "twiddle factor type"=w477) -> (w475:T2)  [unwired: 1 in]
            }
          }
        }
      }
      n220 = case "stage 7" shown="True" FALSE {
        tunnel: w59 -> [w378 w388]
        tunnel: [w378 w387] -> w55
        tunnel: w17 -> [_ w386]
        tunnel: w35 -> [_ w385]
        tunnel: [_ w384] -> w58
        tunnel: [_ w383] -> w57
        tunnel: [_ w382] -> w56
        tunnel: w16 -> [_ w379]
        frame False {
        }
        frame True {
          n221 = call "stage control 7"("enable"=w386, "frame start in"=w388) -> ("next switch"=w382:bool, "frame start out"=w387:bool, "twid index"=w380:fxp<+,7,7>)  [unwired: 7 in]
          n222 = case "tf 7" shown="0, Default" i16 0 {
            tunnel: w379 -> [w390 w398 w414 w428]
            tunnel: w386 -> [w394 w402 w413 w427]
            tunnel: w385 -> [_ _ w412 w426]
            tunnel: [_ _ w407 w421] -> w384
            tunnel: [w391 w399 w406 w420] -> w383
            tunnel: w380 -> [w389 w397 w405 w419]
            frame 0, Default {
              n223 = call <vilib>:"niFpga wdp fft tf 256 U32.vi"("index"=w389, "enable"=w394) -> ("imag"=w395:fxp<+/-,16,2>, "real"=w396:fxp<+/-,16,2>)  [unwired: 8 in]
              n224 = To Fixed-Point(fixed-point type=w390, number=w396) -> (fixed-point=w393:fxp<+/-,16,2>)
              n225 = To Fixed-Point(fixed-point type=w390, number=w395) -> (fixed-point=w392:fxp<+/-,16,2>)
              n226 = Bundle("twiddle factor type"=w393, "twiddle factor type"=w392) -> (w391:T2)  [unwired: 1 in]
            }
            frame 1 {
              n227 = call <vilib>:"niFpga wdp fft tf 256 U64.vi"("index"=w397, "enable"=w402) -> ("imag"=w403:fxp<+/-,32,2>, "real"=w404:fxp<+/-,32,2>)  [unwired: 8 in]
              n228 = To Fixed-Point(fixed-point type=w398, number=w404) -> (fixed-point=w401:fxp<+/-,16,2>)
              n229 = To Fixed-Point(fixed-point type=w398, number=w403) -> (fixed-point=w400:fxp<+/-,16,2>)
              n230 = Bundle("twiddle factor type"=w401, "twiddle factor type"=w400) -> (w399:T2)  [unwired: 1 in]
            }
            frame 2 {
              n231 = call <vilib>:"niFpga wdp fft tf 256 U32.vi"("index"=w405, "enable"=w412) -> ("imag"=w416:fxp<+/-,16,2>, "real"=w417:fxp<+/-,16,2>)  [unwired: 8 in]
              n232 = call <vilib>:"niFpga wdp fft tf 256 U32.vi"("index"=w405, "enable"=w413) -> ("imag"=w415:fxp<+/-,16,2>, "real"=w418:fxp<+/-,16,2>)  [unwired: 8 in]
              n233 = To Fixed-Point(fixed-point type=w414, number=w417) -> (fixed-point=w411:fxp<+/-,16,2>)
              n234 = To Fixed-Point(fixed-point type=w414, number=w416) -> (fixed-point=w410:fxp<+/-,16,2>)
              n235 = To Fixed-Point(fixed-point type=w414, number=w418) -> (fixed-point=w409:fxp<+/-,16,2>)
              n236 = To Fixed-Point(fixed-point type=w414, number=w415) -> (fixed-point=w408:fxp<+/-,16,2>)
              n237 = Bundle("twiddle factor type"=w411, "twiddle factor type"=w410) -> (w407:T2)  [unwired: 1 in]
              n238 = Bundle("twiddle factor type"=w409, "twiddle factor type"=w408) -> (w406:T2)  [unwired: 1 in]
            }
            frame 3 {
              n239 = call <vilib>:"niFpga wdp fft tf 256 U64.vi"("index"=w419, "enable"=w426) -> ("imag"=w430:fxp<+/-,32,2>, "real"=w431:fxp<+/-,32,2>)  [unwired: 8 in]
              n240 = call <vilib>:"niFpga wdp fft tf 256 U64.vi"("index"=w419, "enable"=w427) -> ("imag"=w429:fxp<+/-,32,2>, "real"=w432:fxp<+/-,32,2>)  [unwired: 8 in]
              n241 = To Fixed-Point(fixed-point type=w428, number=w431) -> (fixed-point=w425:fxp<+/-,16,2>)
              n242 = To Fixed-Point(fixed-point type=w428, number=w430) -> (fixed-point=w424:fxp<+/-,16,2>)
              n243 = To Fixed-Point(fixed-point type=w428, number=w432) -> (fixed-point=w423:fxp<+/-,16,2>)
              n244 = To Fixed-Point(fixed-point type=w428, number=w429) -> (fixed-point=w422:fxp<+/-,16,2>)
              n245 = Bundle("twiddle factor type"=w425, "twiddle factor type"=w424) -> (w421:T2)  [unwired: 1 in]
              n246 = Bundle("twiddle factor type"=w423, "twiddle factor type"=w422) -> (w420:T2)  [unwired: 1 in]
            }
          }
        }
      }
      n247 = case "stage 6" shown="True" FALSE {
        tunnel: w55 -> [w323 w333]
        tunnel: [w323 w332] -> w51
        tunnel: w17 -> [_ w331]
        tunnel: w35 -> [_ w330]
        tunnel: [_ w329] -> w54
        tunnel: [_ w328] -> w53
        tunnel: [_ w327] -> w52
        tunnel: w16 -> [_ w324]
        frame False {
        }
        frame True {
          n248 = call "stage control 6"("enable"=w331, "frame start in"=w333) -> ("next switch"=w327:bool, "frame start out"=w332:bool, "twid index"=w325:fxp<+,6,6>)  [unwired: 7 in]
          n249 = case "tf 6" shown="0, Default" i16 0 {
            tunnel: w324 -> [w335 w343 w359 w373]
            tunnel: w331 -> [w339 w347 w358 w372]
            tunnel: w330 -> [_ _ w357 w371]
            tunnel: [_ _ w352 w366] -> w329
            tunnel: [w336 w344 w351 w365] -> w328
            tunnel: w325 -> [w334 w342 w350 w364]
            frame 0, Default {
              n250 = call <vilib>:"niFpga wdp fft tf 128 U32.vi"("index"=w334, "enable"=w339) -> ("imag"=w340:fxp<+/-,16,2>, "real"=w341:fxp<+/-,16,2>)  [unwired: 8 in]
              n251 = To Fixed-Point(fixed-point type=w335, number=w341) -> (fixed-point=w338:fxp<+/-,16,2>)
              n252 = To Fixed-Point(fixed-point type=w335, number=w340) -> (fixed-point=w337:fxp<+/-,16,2>)
              n253 = Bundle("twiddle factor type"=w338, "twiddle factor type"=w337) -> (w336:T2)  [unwired: 1 in]
            }
            frame 1 {
              n254 = call <vilib>:"niFpga wdp fft tf 128 U64.vi"("index"=w342, "enable"=w347) -> ("imag"=w348:fxp<+/-,32,2>, "real"=w349:fxp<+/-,32,2>)  [unwired: 8 in]
              n255 = To Fixed-Point(fixed-point type=w343, number=w349) -> (fixed-point=w346:fxp<+/-,16,2>)
              n256 = To Fixed-Point(fixed-point type=w343, number=w348) -> (fixed-point=w345:fxp<+/-,16,2>)
              n257 = Bundle("twiddle factor type"=w346, "twiddle factor type"=w345) -> (w344:T2)  [unwired: 1 in]
            }
            frame 2 {
              n258 = call <vilib>:"niFpga wdp fft tf 128 U32.vi"("index"=w350, "enable"=w357) -> ("imag"=w361:fxp<+/-,16,2>, "real"=w362:fxp<+/-,16,2>)  [unwired: 8 in]
              n259 = call <vilib>:"niFpga wdp fft tf 128 U32.vi"("index"=w350, "enable"=w358) -> ("imag"=w360:fxp<+/-,16,2>, "real"=w363:fxp<+/-,16,2>)  [unwired: 8 in]
              n260 = To Fixed-Point(fixed-point type=w359, number=w362) -> (fixed-point=w356:fxp<+/-,16,2>)
              n261 = To Fixed-Point(fixed-point type=w359, number=w361) -> (fixed-point=w355:fxp<+/-,16,2>)
              n262 = To Fixed-Point(fixed-point type=w359, number=w363) -> (fixed-point=w354:fxp<+/-,16,2>)
              n263 = To Fixed-Point(fixed-point type=w359, number=w360) -> (fixed-point=w353:fxp<+/-,16,2>)
              n264 = Bundle("twiddle factor type"=w356, "twiddle factor type"=w355) -> (w352:T2)  [unwired: 1 in]
              n265 = Bundle("twiddle factor type"=w354, "twiddle factor type"=w353) -> (w351:T2)  [unwired: 1 in]
            }
            frame 3 {
              n266 = call <vilib>:"niFpga wdp fft tf 128 U64.vi"("index"=w364, "enable"=w371) -> ("imag"=w375:fxp<+/-,32,2>, "real"=w376:fxp<+/-,32,2>)  [unwired: 8 in]
              n267 = call <vilib>:"niFpga wdp fft tf 128 U64.vi"("index"=w364, "enable"=w372) -> ("imag"=w374:fxp<+/-,32,2>, "real"=w377:fxp<+/-,32,2>)  [unwired: 8 in]
              n268 = To Fixed-Point(fixed-point type=w373, number=w376) -> (fixed-point=w370:fxp<+/-,16,2>)
              n269 = To Fixed-Point(fixed-point type=w373, number=w375) -> (fixed-point=w369:fxp<+/-,16,2>)
              n270 = To Fixed-Point(fixed-point type=w373, number=w377) -> (fixed-point=w368:fxp<+/-,16,2>)
              n271 = To Fixed-Point(fixed-point type=w373, number=w374) -> (fixed-point=w367:fxp<+/-,16,2>)
              n272 = Bundle("twiddle factor type"=w370, "twiddle factor type"=w369) -> (w366:T2)  [unwired: 1 in]
              n273 = Bundle("twiddle factor type"=w368, "twiddle factor type"=w367) -> (w365:T2)  [unwired: 1 in]
            }
          }
        }
      }
      n274 = case "stage 5" shown="True" FALSE {
        tunnel: w51 -> [w268 w278]
        tunnel: [w268 w277] -> w47
        tunnel: w17 -> [_ w276]
        tunnel: w35 -> [_ w275]
        tunnel: [_ w274] -> w50
        tunnel: [_ w273] -> w49
        tunnel: [_ w272] -> w48
        tunnel: w16 -> [_ w269]
        frame False {
        }
        frame True {
          n275 = call "stage control 5"("enable"=w276, "frame start in"=w278) -> ("next switch"=w272:bool, "frame start out"=w277:bool, "twid index"=w270:fxp<+,5,5>)  [unwired: 7 in]
          n276 = case "tf 5" shown="0, Default" i16 0 {
            tunnel: w269 -> [w280 w288 w304 w318]
            tunnel: w276 -> [w284 w292 w303 w317]
            tunnel: w275 -> [_ _ w302 w316]
            tunnel: [_ _ w297 w311] -> w274
            tunnel: [w281 w289 w296 w310] -> w273
            tunnel: w270 -> [w279 w287 w295 w309]
            frame 0, Default {
              n277 = call <vilib>:"niFpga wdp fft tf 64 U32.vi"("index"=w279, "enable"=w284) -> ("imag"=w285:fxp<+/-,16,2>, "real"=w286:fxp<+/-,16,2>)  [unwired: 8 in]
              n278 = To Fixed-Point(fixed-point type=w280, number=w286) -> (fixed-point=w283:fxp<+/-,16,2>)
              n279 = To Fixed-Point(fixed-point type=w280, number=w285) -> (fixed-point=w282:fxp<+/-,16,2>)
              n280 = Bundle("twiddle factor type"=w283, "twiddle factor type"=w282) -> (w281:T2)  [unwired: 1 in]
            }
            frame 1 {
              n281 = call <vilib>:"niFpga wdp fft tf 64 U64.vi"("index"=w287, "enable"=w292) -> ("imag"=w293:fxp<+/-,32,2>, "real"=w294:fxp<+/-,32,2>)  [unwired: 8 in]
              n282 = To Fixed-Point(fixed-point type=w288, number=w294) -> (fixed-point=w291:fxp<+/-,16,2>)
              n283 = To Fixed-Point(fixed-point type=w288, number=w293) -> (fixed-point=w290:fxp<+/-,16,2>)
              n284 = Bundle("twiddle factor type"=w291, "twiddle factor type"=w290) -> (w289:T2)  [unwired: 1 in]
            }
            frame 2 {
              n285 = call <vilib>:"niFpga wdp fft tf 64 U32.vi"("index"=w295, "enable"=w302) -> ("imag"=w306:fxp<+/-,16,2>, "real"=w307:fxp<+/-,16,2>)  [unwired: 8 in]
              n286 = call <vilib>:"niFpga wdp fft tf 64 U32.vi"("index"=w295, "enable"=w303) -> ("imag"=w305:fxp<+/-,16,2>, "real"=w308:fxp<+/-,16,2>)  [unwired: 8 in]
              n287 = To Fixed-Point(fixed-point type=w304, number=w307) -> (fixed-point=w301:fxp<+/-,16,2>)
              n288 = To Fixed-Point(fixed-point type=w304, number=w306) -> (fixed-point=w300:fxp<+/-,16,2>)
              n289 = To Fixed-Point(fixed-point type=w304, number=w308) -> (fixed-point=w299:fxp<+/-,16,2>)
              n290 = To Fixed-Point(fixed-point type=w304, number=w305) -> (fixed-point=w298:fxp<+/-,16,2>)
              n291 = Bundle("twiddle factor type"=w301, "twiddle factor type"=w300) -> (w297:T2)  [unwired: 1 in]
              n292 = Bundle("twiddle factor type"=w299, "twiddle factor type"=w298) -> (w296:T2)  [unwired: 1 in]
            }
            frame 3 {
              n293 = call <vilib>:"niFpga wdp fft tf 64 U64.vi"("index"=w309, "enable"=w316) -> ("imag"=w320:fxp<+/-,32,2>, "real"=w321:fxp<+/-,32,2>)  [unwired: 8 in]
              n294 = call <vilib>:"niFpga wdp fft tf 64 U64.vi"("index"=w309, "enable"=w317) -> ("imag"=w319:fxp<+/-,32,2>, "real"=w322:fxp<+/-,32,2>)  [unwired: 8 in]
              n295 = To Fixed-Point(fixed-point type=w318, number=w321) -> (fixed-point=w315:fxp<+/-,16,2>)
              n296 = To Fixed-Point(fixed-point type=w318, number=w320) -> (fixed-point=w314:fxp<+/-,16,2>)
              n297 = To Fixed-Point(fixed-point type=w318, number=w322) -> (fixed-point=w313:fxp<+/-,16,2>)
              n298 = To Fixed-Point(fixed-point type=w318, number=w319) -> (fixed-point=w312:fxp<+/-,16,2>)
              n299 = Bundle("twiddle factor type"=w315, "twiddle factor type"=w314) -> (w311:T2)  [unwired: 1 in]
              n300 = Bundle("twiddle factor type"=w313, "twiddle factor type"=w312) -> (w310:T2)  [unwired: 1 in]
            }
          }
        }
      }
      n301 = case "stage 4" shown="True" FALSE {
        tunnel: w47 -> [w213 w223]
        tunnel: [w213 w222] -> w43
        tunnel: w17 -> [_ w221]
        tunnel: w35 -> [_ w220]
        tunnel: [_ w219] -> w46
        tunnel: [_ w218] -> w45
        tunnel: [_ w217] -> w44
        tunnel: w16 -> [_ w214]
        frame False {
        }
        frame True {
          n302 = call "stage control 4"("enable"=w221, "frame start in"=w223) -> ("next switch"=w217:bool, "frame start out"=w222:bool, "twid index"=w215:fxp<+,4,4>)  [unwired: 7 in]
          n303 = case "tf 4" shown="0, Default" i16 0 {
            tunnel: w214 -> [w225 w233 w249 w263]
            tunnel: w221 -> [w229 w237 w248 w262]
            tunnel: w220 -> [_ _ w247 w261]
            tunnel: [_ _ w242 w256] -> w219
            tunnel: [w226 w234 w241 w255] -> w218
            tunnel: w215 -> [w224 w232 w240 w254]
            frame 0, Default {
              n304 = call <vilib>:"niFpga wdp fft tf 32 U32.vi"("index"=w224, "enable"=w229) -> ("imag"=w230:fxp<+/-,16,2>, "real"=w231:fxp<+/-,16,2>)  [unwired: 8 in]
              n305 = To Fixed-Point(fixed-point type=w225, number=w231) -> (fixed-point=w228:fxp<+/-,16,2>)
              n306 = To Fixed-Point(fixed-point type=w225, number=w230) -> (fixed-point=w227:fxp<+/-,16,2>)
              n307 = Bundle("twiddle factor type"=w228, "twiddle factor type"=w227) -> (w226:T2)  [unwired: 1 in]
            }
            frame 1 {
              n308 = call <vilib>:"niFpga wdp fft tf 32 U64.vi"("index"=w232, "enable"=w237) -> ("imag"=w238:fxp<+/-,32,2>, "real"=w239:fxp<+/-,32,2>)  [unwired: 8 in]
              n309 = To Fixed-Point(fixed-point type=w233, number=w239) -> (fixed-point=w236:fxp<+/-,16,2>)
              n310 = To Fixed-Point(fixed-point type=w233, number=w238) -> (fixed-point=w235:fxp<+/-,16,2>)
              n311 = Bundle("twiddle factor type"=w236, "twiddle factor type"=w235) -> (w234:T2)  [unwired: 1 in]
            }
            frame 2 {
              n312 = call <vilib>:"niFpga wdp fft tf 32 U32.vi"("index"=w240, "enable"=w247) -> ("imag"=w251:fxp<+/-,16,2>, "real"=w252:fxp<+/-,16,2>)  [unwired: 8 in]
              n313 = call <vilib>:"niFpga wdp fft tf 32 U32.vi"("index"=w240, "enable"=w248) -> ("imag"=w250:fxp<+/-,16,2>, "real"=w253:fxp<+/-,16,2>)  [unwired: 8 in]
              n314 = To Fixed-Point(fixed-point type=w249, number=w252) -> (fixed-point=w246:fxp<+/-,16,2>)
              n315 = To Fixed-Point(fixed-point type=w249, number=w251) -> (fixed-point=w245:fxp<+/-,16,2>)
              n316 = To Fixed-Point(fixed-point type=w249, number=w253) -> (fixed-point=w244:fxp<+/-,16,2>)
              n317 = To Fixed-Point(fixed-point type=w249, number=w250) -> (fixed-point=w243:fxp<+/-,16,2>)
              n318 = Bundle("twiddle factor type"=w246, "twiddle factor type"=w245) -> (w242:T2)  [unwired: 1 in]
              n319 = Bundle("twiddle factor type"=w244, "twiddle factor type"=w243) -> (w241:T2)  [unwired: 1 in]
            }
            frame 3 {
              n320 = call <vilib>:"niFpga wdp fft tf 32 U64.vi"("index"=w254, "enable"=w261) -> ("imag"=w265:fxp<+/-,32,2>, "real"=w266:fxp<+/-,32,2>)  [unwired: 8 in]
              n321 = call <vilib>:"niFpga wdp fft tf 32 U64.vi"("index"=w254, "enable"=w262) -> ("imag"=w264:fxp<+/-,32,2>, "real"=w267:fxp<+/-,32,2>)  [unwired: 8 in]
              n322 = To Fixed-Point(fixed-point type=w263, number=w266) -> (fixed-point=w260:fxp<+/-,16,2>)
              n323 = To Fixed-Point(fixed-point type=w263, number=w265) -> (fixed-point=w259:fxp<+/-,16,2>)
              n324 = To Fixed-Point(fixed-point type=w263, number=w267) -> (fixed-point=w258:fxp<+/-,16,2>)
              n325 = To Fixed-Point(fixed-point type=w263, number=w264) -> (fixed-point=w257:fxp<+/-,16,2>)
              n326 = Bundle("twiddle factor type"=w260, "twiddle factor type"=w259) -> (w256:T2)  [unwired: 1 in]
              n327 = Bundle("twiddle factor type"=w258, "twiddle factor type"=w257) -> (w255:T2)  [unwired: 1 in]
            }
          }
        }
      }
      n328 = case "stage 3" shown="True" FALSE {
        tunnel: w43 -> [w158 w168]
        tunnel: [w158 w167] -> w39
        tunnel: w17 -> [_ w166]
        tunnel: w35 -> [_ w165]
        tunnel: [_ w164] -> w42
        tunnel: [_ w163] -> w41
        tunnel: [_ w162] -> w40
        tunnel: w16 -> [_ w159]
        frame False {
        }
        frame True {
          n329 = call "stage control 3"("enable"=w166, "frame start in"=w168) -> ("next switch"=w162:bool, "frame start out"=w167:bool, "twid index"=w160:fxp<+,3,3>)  [unwired: 7 in]
          n330 = case "tf 3" shown="0, Default" i16 0 {
            tunnel: w159 -> [w170 w178 w194 w208]
            tunnel: w166 -> [w174 w182 w193 w207]
            tunnel: w165 -> [_ _ w192 w206]
            tunnel: [_ _ w187 w201] -> w164
            tunnel: [w171 w179 w186 w200] -> w163
            tunnel: w160 -> [w169 w177 w185 w199]
            frame 0, Default {
              n331 = call <vilib>:"niFpga wdp fft tf 16 U32.vi"("index"=w169, "enable"=w174) -> ("imag"=w175:fxp<+/-,16,2>, "real"=w176:fxp<+/-,16,2>)  [unwired: 8 in]
              n332 = To Fixed-Point(fixed-point type=w170, number=w176) -> (fixed-point=w173:fxp<+/-,16,2>)
              n333 = To Fixed-Point(fixed-point type=w170, number=w175) -> (fixed-point=w172:fxp<+/-,16,2>)
              n334 = Bundle("twiddle factor type"=w173, "twiddle factor type"=w172) -> (w171:T2)  [unwired: 1 in]
            }
            frame 1 {
              n335 = call <vilib>:"niFpga wdp fft tf 16 U64.vi"("index"=w177, "enable"=w182) -> ("imag"=w183:fxp<+/-,32,2>, "real"=w184:fxp<+/-,32,2>)  [unwired: 8 in]
              n336 = To Fixed-Point(fixed-point type=w178, number=w184) -> (fixed-point=w181:fxp<+/-,16,2>)
              n337 = To Fixed-Point(fixed-point type=w178, number=w183) -> (fixed-point=w180:fxp<+/-,16,2>)
              n338 = Bundle("twiddle factor type"=w181, "twiddle factor type"=w180) -> (w179:T2)  [unwired: 1 in]
            }
            frame 2 {
              n339 = call <vilib>:"niFpga wdp fft tf 16 U32.vi"("index"=w185, "enable"=w192) -> ("imag"=w196:fxp<+/-,16,2>, "real"=w197:fxp<+/-,16,2>)  [unwired: 8 in]
              n340 = call <vilib>:"niFpga wdp fft tf 16 U32.vi"("index"=w185, "enable"=w193) -> ("imag"=w195:fxp<+/-,16,2>, "real"=w198:fxp<+/-,16,2>)  [unwired: 8 in]
              n341 = To Fixed-Point(fixed-point type=w194, number=w197) -> (fixed-point=w191:fxp<+/-,16,2>)
              n342 = To Fixed-Point(fixed-point type=w194, number=w196) -> (fixed-point=w190:fxp<+/-,16,2>)
              n343 = To Fixed-Point(fixed-point type=w194, number=w198) -> (fixed-point=w189:fxp<+/-,16,2>)
              n344 = To Fixed-Point(fixed-point type=w194, number=w195) -> (fixed-point=w188:fxp<+/-,16,2>)
              n345 = Bundle("twiddle factor type"=w191, "twiddle factor type"=w190) -> (w187:T2)  [unwired: 1 in]
              n346 = Bundle("twiddle factor type"=w189, "twiddle factor type"=w188) -> (w186:T2)  [unwired: 1 in]
            }
            frame 3 {
              n347 = call <vilib>:"niFpga wdp fft tf 16 U64.vi"("index"=w199, "enable"=w206) -> ("imag"=w210:fxp<+/-,32,2>, "real"=w211:fxp<+/-,32,2>)  [unwired: 8 in]
              n348 = call <vilib>:"niFpga wdp fft tf 16 U64.vi"("index"=w199, "enable"=w207) -> ("imag"=w209:fxp<+/-,32,2>, "real"=w212:fxp<+/-,32,2>)  [unwired: 8 in]
              n349 = To Fixed-Point(fixed-point type=w208, number=w211) -> (fixed-point=w205:fxp<+/-,16,2>)
              n350 = To Fixed-Point(fixed-point type=w208, number=w210) -> (fixed-point=w204:fxp<+/-,16,2>)
              n351 = To Fixed-Point(fixed-point type=w208, number=w212) -> (fixed-point=w203:fxp<+/-,16,2>)
              n352 = To Fixed-Point(fixed-point type=w208, number=w209) -> (fixed-point=w202:fxp<+/-,16,2>)
              n353 = Bundle("twiddle factor type"=w205, "twiddle factor type"=w204) -> (w201:T2)  [unwired: 1 in]
              n354 = Bundle("twiddle factor type"=w203, "twiddle factor type"=w202) -> (w200:T2)  [unwired: 1 in]
            }
          }
        }
      }
      n355 = case "stage 2" shown="True" FALSE {
        tunnel: w39 -> [w103 w113]
        tunnel: [w103 w112] -> w34
        tunnel: w17 -> [_ w111]
        tunnel: w35 -> [_ w110]
        tunnel: [_ w109] -> w38
        tunnel: [_ w108] -> w37
        tunnel: [_ w107] -> w36
        tunnel: w16 -> [_ w104]
        frame False {
        }
        frame True {
          n356 = call "stage control 2"("enable"=w111, "frame start in"=w113) -> ("next switch"=w107:bool, "frame start out"=w112:bool, "twid index"=w105:fxp<+,2,2>)  [unwired: 7 in]
          n357 = case "tf 2" shown="0, Default" i16 0 {
            tunnel: w104 -> [w115 w123 w139 w153]
            tunnel: w111 -> [w119 w127 w138 w152]
            tunnel: w110 -> [_ _ w137 w151]
            tunnel: [_ _ w132 w146] -> w109
            tunnel: [w116 w124 w131 w145] -> w108
            tunnel: w105 -> [w114 w122 w130 w144]
            frame 0, Default {
              n358 = call <vilib>:"niFpga wdp fft tf 8 U32.vi"("index"=w114, "enable"=w119) -> ("imag"=w120:fxp<+/-,16,2>, "real"=w121:fxp<+/-,16,2>)  [unwired: 8 in]
              n359 = To Fixed-Point(fixed-point type=w115, number=w121) -> (fixed-point=w118:fxp<+/-,16,2>)
              n360 = To Fixed-Point(fixed-point type=w115, number=w120) -> (fixed-point=w117:fxp<+/-,16,2>)
              n361 = Bundle("twiddle factor type"=w118, "twiddle factor type"=w117) -> (w116:T2)  [unwired: 1 in]
            }
            frame 1 {
              n362 = call <vilib>:"niFpga wdp fft tf 8 U64.vi"("index"=w122, "enable"=w127) -> ("imag"=w128:fxp<+/-,32,2>, "real"=w129:fxp<+/-,32,2>)  [unwired: 8 in]
              n363 = To Fixed-Point(fixed-point type=w123, number=w129) -> (fixed-point=w126:fxp<+/-,16,2>)
              n364 = To Fixed-Point(fixed-point type=w123, number=w128) -> (fixed-point=w125:fxp<+/-,16,2>)
              n365 = Bundle("twiddle factor type"=w126, "twiddle factor type"=w125) -> (w124:T2)  [unwired: 1 in]
            }
            frame 2 {
              n366 = call <vilib>:"niFpga wdp fft tf 8 U32.vi"("index"=w130, "enable"=w137) -> ("imag"=w141:fxp<+/-,16,2>, "real"=w142:fxp<+/-,16,2>)  [unwired: 8 in]
              n367 = call <vilib>:"niFpga wdp fft tf 8 U32.vi"("index"=w130, "enable"=w138) -> ("imag"=w140:fxp<+/-,16,2>, "real"=w143:fxp<+/-,16,2>)  [unwired: 8 in]
              n368 = To Fixed-Point(fixed-point type=w139, number=w142) -> (fixed-point=w136:fxp<+/-,16,2>)
              n369 = To Fixed-Point(fixed-point type=w139, number=w141) -> (fixed-point=w135:fxp<+/-,16,2>)
              n370 = To Fixed-Point(fixed-point type=w139, number=w143) -> (fixed-point=w134:fxp<+/-,16,2>)
              n371 = To Fixed-Point(fixed-point type=w139, number=w140) -> (fixed-point=w133:fxp<+/-,16,2>)
              n372 = Bundle("twiddle factor type"=w136, "twiddle factor type"=w135) -> (w132:T2)  [unwired: 1 in]
              n373 = Bundle("twiddle factor type"=w134, "twiddle factor type"=w133) -> (w131:T2)  [unwired: 1 in]
            }
            frame 3 {
              n374 = call <vilib>:"niFpga wdp fft tf 8 U64.vi"("index"=w144, "enable"=w151) -> ("imag"=w155:fxp<+/-,32,2>, "real"=w156:fxp<+/-,32,2>)  [unwired: 8 in]
              n375 = call <vilib>:"niFpga wdp fft tf 8 U64.vi"("index"=w144, "enable"=w152) -> ("imag"=w154:fxp<+/-,32,2>, "real"=w157:fxp<+/-,32,2>)  [unwired: 8 in]
              n376 = To Fixed-Point(fixed-point type=w153, number=w156) -> (fixed-point=w150:fxp<+/-,16,2>)
              n377 = To Fixed-Point(fixed-point type=w153, number=w155) -> (fixed-point=w149:fxp<+/-,16,2>)
              n378 = To Fixed-Point(fixed-point type=w153, number=w157) -> (fixed-point=w148:fxp<+/-,16,2>)
              n379 = To Fixed-Point(fixed-point type=w153, number=w154) -> (fixed-point=w147:fxp<+/-,16,2>)
              n380 = Bundle("twiddle factor type"=w150, "twiddle factor type"=w149) -> (w146:T2)  [unwired: 1 in]
              n381 = Bundle("twiddle factor type"=w148, "twiddle factor type"=w147) -> (w145:T2)  [unwired: 1 in]
            }
          }
        }
      }
      n382 = case "stage 1" shown="True" FALSE {
        tunnel: w34 -> [w95 w102]
        tunnel: [_ w101] -> w33
        tunnel: [_ w98] -> w32
        tunnel: w17 -> [_ w97]
        tunnel: [w95 w96] -> w14
        frame False {
        }
        frame True {
          n383 = call "stage control 1"("enable"=w97, "frame start in"=w102) -> ("next switch"=w101:bool, "frame start out"=w96:bool, "twid index"=w99:fxp<+,1,1>)  [unwired: 7 in]
          n384 = Equal To 0?(x=w99) -> (x = 0?=w100:bool)
          n385 = feedback #2() -> (w98:bool)  [unwired: 1 in]
          n386 = feedback-in #2(w100, w97) -> ()
        }
      }
      n387 = Build Array "Build Array tf 1"(w38, w42, w46, w50, w54, w58, w62, w66, w70, w74, w78, w82, w86, w90) -> (w92:T1)
      n388 = Build Array "Build Array tf"(w37, w41, w45, w49, w53, w57, w61, w65, w69, w73, w77, w81, w85, w89) -> (w93:T1)
      n389 = Build Array "Build Array switch"(w33, w36, w40, w44, w48, w52, w56, w60, w64, w68, w72, w76, w80, w84, w88) -> (w94:bool[])
    }
  }
  "frame start" <- w5
  "switch" <- w9
  "index=0?" <- w1
  "twiddle factors" <- w8
  "twiddle factors 1" <- w7
